vi "PH_IEEE1394Camera.set ROI Pair.vi"(2 "Lower Limit":u32, 3 "Input 2":u32, 4 "Input 1":u32, 5 "Upper Limit":u32) -> (0 "Lower Output":u32, 1 "Higher Output":u32)   [LabVIEW 2014, in "PH_IEEE1394Camera.lvlib"]
doc: "The Output of this VI is a lower and a higher number. They are calculated out of Input 1 and 2, they are limited by the lower and higher limits (which are includet) and differ by at least 1."
uses:
  PH_IEEE1394Camera.lvlib
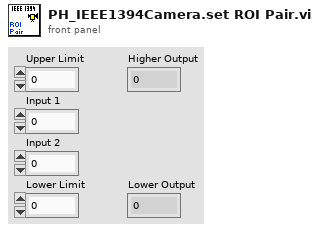
[diagram p1: front panel]
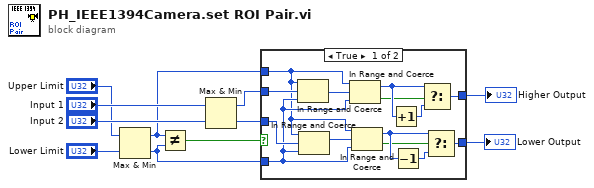
[diagram p0: block diagram]
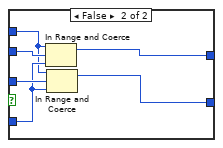
[diagram p2: hidden frame]
diagram:
  n1 = Max & Min(x="Upper Limit", y="Lower Limit") -> (max(x,y)=w2:u32, min(x,y)=w3:u32)
  n2 = Not Equal?(x=w2, y=w3) -> (x != y?=w1:bool)
  n3 = Max & Min(x="Input 1", y="Input 2") -> (max(x,y)=w7:u32, min(x,y)=w9:u32)
  n4 = case shown="True" w1 {
    tunnel: w9 -> [w25 w31]
    tunnel: [w23 w30] -> w8
    tunnel: w7 -> [w24 w29]
    tunnel: [w20 w28] -> w6
    tunnel: w3 -> [w17 w27]
    tunnel: w2 -> [w16 w26]
    frame True {
      n5 = In Range and Coerce(upper limit=w16, x=w24, lower limit=w17) -> (coerced(x)=w19:u32)  [unwired: 1 out]
      n6 = In Range and Coerce(upper limit=w16, x=w25, lower limit=w17) -> (coerced(x)=w15:u32)  [unwired: 1 out]
      n7 = In Range and Coerce(upper limit=w16, x=w19, lower limit=w17) -> (coerced(x)=w18:u32, In Range?=w12:bool)
      n8 = In Range and Coerce(upper limit=w16, x=w15, lower limit=w17) -> (coerced(x)=w14:u32, In Range?=w13:bool)
      n9 = Increment(x=w18) -> (x+1=w21:u32)
      n10 = Decrement(x=w14) -> (x-1=w22:u32)
      n11 = Select(t=w18, s=w12, f=w21) -> (s? t:f=w20:u32)
      n12 = Select(t=w14, s=w13, f=w22) -> (s? t:f=w23:u32)
    }
    frame False {
      n13 = In Range and Coerce(upper limit=w26, x=w29, lower limit=w27) -> (coerced(x)=w28:u32)  [unwired: 1 out]
      n14 = In Range and Coerce(upper limit=w26, x=w31, lower limit=w27) -> (coerced(x)=w30:u32)  [unwired: 1 out]
    }
  }
  "Higher Output" <- w6
  "Lower Output" <- w8
